vi "GetLimsTestSteps.vi"(8 "error in (no error)":errorcluster, 10 "Test-id":i32, 11 "ByteGSAPIBase in":refnum<class "ByteGSAPIBase.lvclass">) -> (0 "error out":errorcluster, 2 "Test Steps List":T1[](array[typedef]), 3 "ByteGSAPIBase out":refnum<class "ByteGSAPIBase.lvclass">)   [LabVIEW 2019, in "ByteGSWebAPI.lvlib" / "ByteGSAPIBase.lvclass"]
doc: "Get list of steps based on Test-id"
uses:
  ByteGSAPIBase.lvclass
  TypeDef/Step.ctl
  TypeDef/Asset.ctl
  ByteGSAPIBase.lvclass/ByteGSAPIBase.ctl
  <vilib>/Bytelabs/ByteREST/ByteRESTClass/ByteRESTBase/RESTBase.lvclass
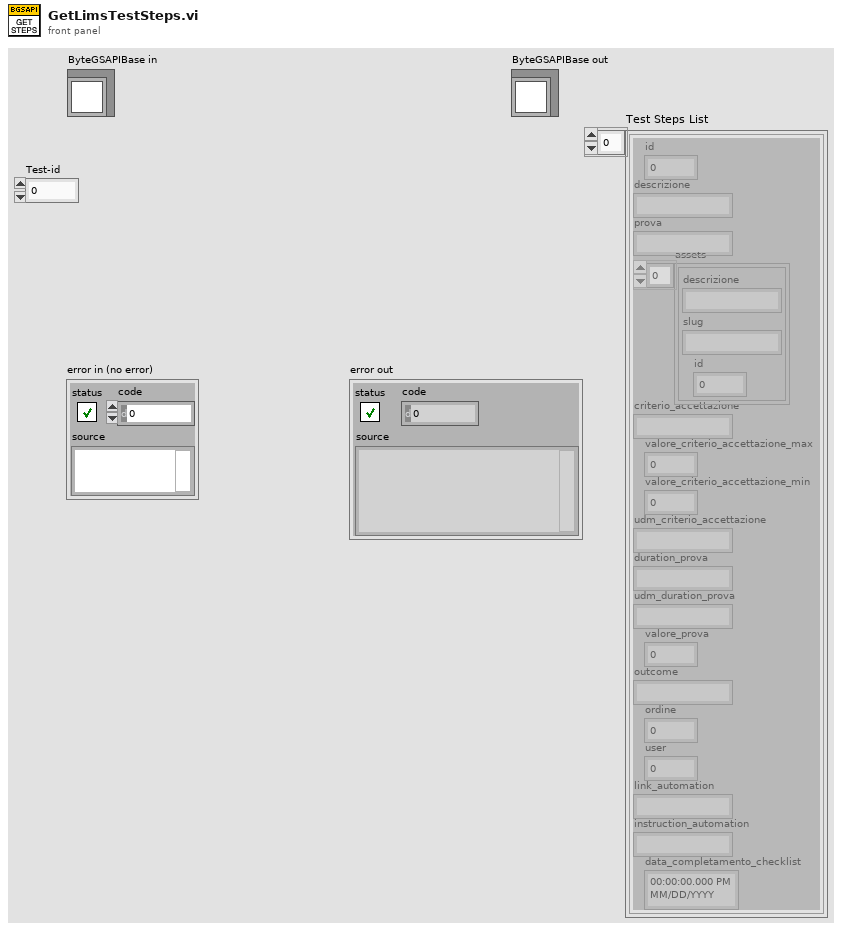
[diagram p1: front panel]
types:
  T1 = typedef "ByteGSWebAPI.lvlib/ByteGSAPIBase.lvclass/Step.ctl" = cluster{"id":i32, "descrizione":string, "prova":string, "assets":T2[], "criterio_accettazione":string, "valore_criterio_accettazione_max":dbl, "valore_criterio_accettazione_min":dbl, "udm_criterio_accettazione":string, "duration_prova":string, "udm_duration_prova":string, "valore_prova":dbl, "outcome":string, "ordine":i32, "user":i32, "link_automation":string, "instruction_automation":string, "data_completamento_checklist":timestamp}
  T2 = typedef "ByteGSWebAPI.lvlib/ByteGSAPIBase.lvclass/Asset.ctl" = cluster{"descrizione":string, "slug":string, "id":i32}
  T3 = cluster{"id":i32, "descrizione":string, "prova":string, "assets":T2[], "criterio_accettazione":string, "valore_criterio_accettazione_max":dbl, "valore_criterio_accettazione_min":dbl, "udm_criterio_accettazione":string, "duration_prova":string, "udm_duration_prova":string, "data_completamento_checklist":string, "valore_prova":dbl, "outcome":string, "ordine":i32, "user":i32, "link_automation":string, "instruction_automation":string}[]
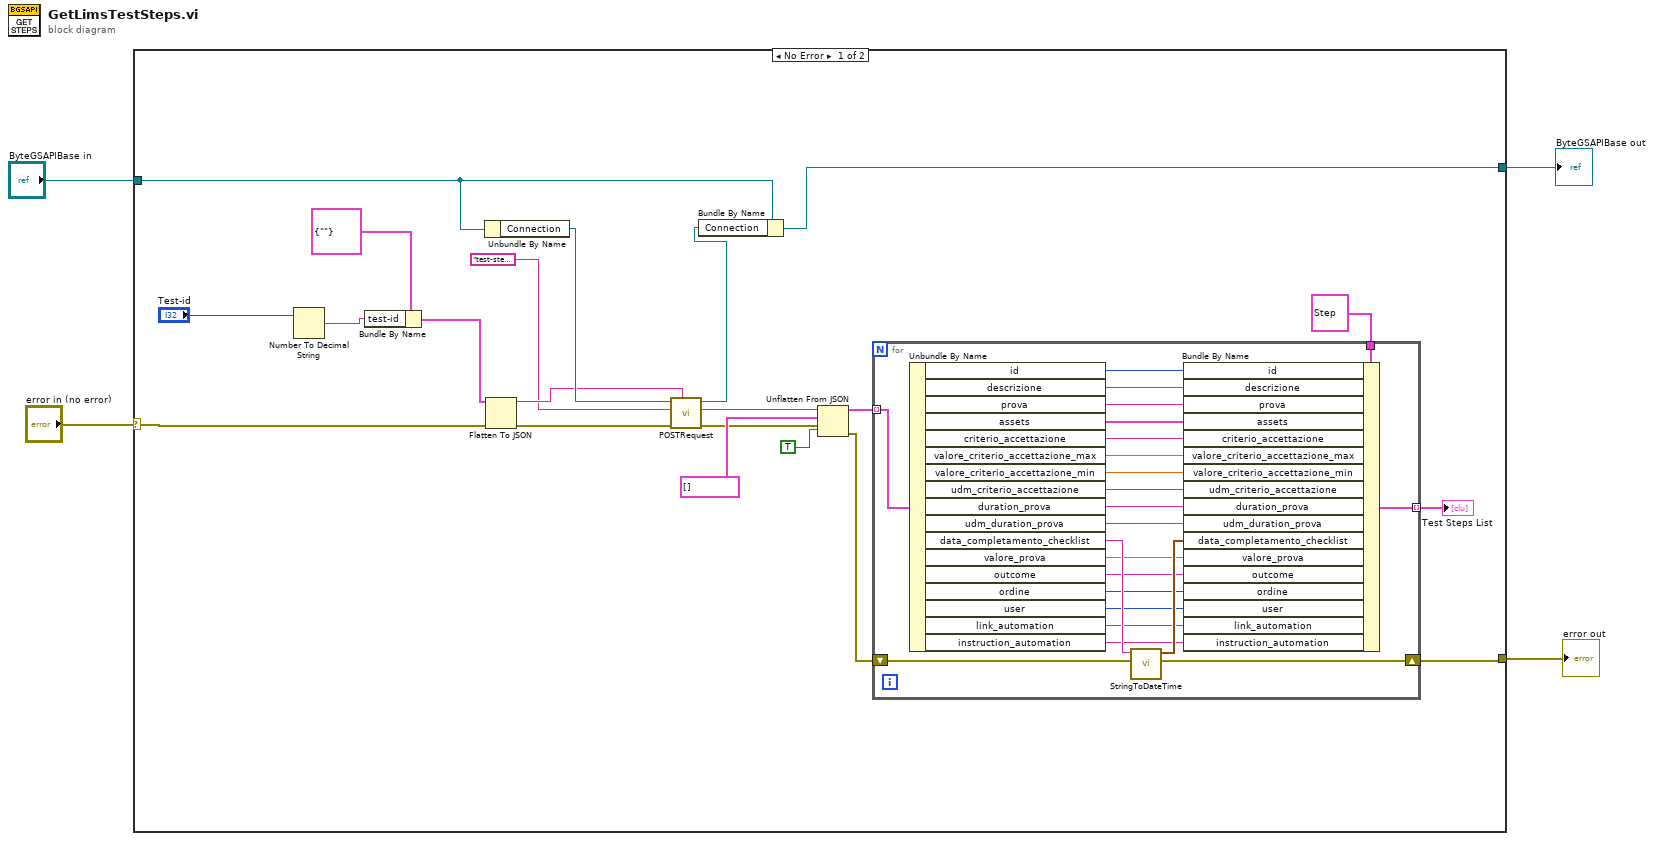
[diagram p0: block diagram]
diagram:
  n1 = case shown="No Error" "error in (no error)" {
    selector: "error in (no error)" -> [w22 w50]
    tunnel: [w7 w50] -> w3
    tunnel: [w23 w49] -> w1
    tunnel: "ByteGSAPIBase in" -> [w14 w49]
    frame No Error {
      n2 = Number To Decimal String(number="Test-id") -> (decimal integer string=w12:string)  [unwired: 1 in]
      n3 = Bundle By Name(cluster=cluster{"test-id":string} {"test-id"=""} ("Request"), "test-id"=w12) -> (w11:cluster{"test-id":string})
      n4 = Unbundle By Name(w14) -> ("Connection"=w25:refnum<class "RESTBase.lvclass">)
      n5 = Flatten To JSON(anything=w11, error in (no error)=w22) -> (JSON string=w20:string, 11:w24:errorcluster)  [unwired: 1 in]
      n6 = call-dynamic "POSTRequest.vi"("Body in"=w20, "error in (no error)"=w24, "Request"="test-step-list", "ByteRESTBase in"=w25) -> ("error out"=w18:errorcluster, "Body"=w16:string, "ByteRESTBase out"=w17:refnum<class "RESTBase.lvclass">)  [unwired: 4 in, 1 out]
      n7 = Bundle By Name(cluster=w14, "Connection"=w17) -> (w23:refnum<class "ByteGSAPIBase.lvclass">)
      n8 = Unflatten From JSON(JSON string=w16, type and defaults=T3 [], default null elements? (F)=TRUE, error in (no error)=w18) -> (value=w10:T3, error out=w8:errorcluster)  [unwired: 3 in]
      n9 = for {
        tunnel: w10 -> [w48] mode=indexing
        tunnel: T1 {"id"=0, "descrizione"="", "prova"="", "assets"=[], "criterio_accettazione"="", "valore_criterio_accettazione_max"=0.0, "valore_criterio_accettazione_min"=0.0, "udm_criterio_accettazione"="", "duration_prova"="", "udm_duration_prova"="", "valore_prova"=0.0, "outcome"="", "ordine"=0, "user"=0, "link_automation"="", "instruction_automation"="", "data_completamento_checklist"=timestamp(0 s since 1904-01-01)} -> [w47]
        shift-right: [w27] -> w7
        shift-left: w8 -> [w28]
        tunnel: [w26] -> w5 mode=indexing
        n10 = Unbundle By Name(w48) -> ("id"=w46:i32, "descrizione"=w45:string, "prova"=w44:string, "assets"=w43:T2[], "criterio_accettazione"=w42:string, "valore_criterio_accettazione_max"=w41:dbl, "valore_criterio_accettazione_min"=w40:dbl, "udm_criterio_accettazione"=w39:string, "duration_prova"=w38:string, "udm_duration_prova"=w37:string, "data_completamento_checklist"=w36:string, "valore_prova"=w34:dbl, "outcome"=w33:string, "ordine"=w32:i32, "user"=w31:i32, "link_automation"=w30:string, "instruction_automation"=w29:string)
        n11 = call "StringToDateTime.vi"("error in (no error)"=w28, "datetime string"=w36) -> ("error out"=w27:errorcluster, "timestamp"=w35:timestamp)  [unwired: 8 in]
        n12 = Bundle By Name(cluster=w47, "id"=w46, "descrizione"=w45, "prova"=w44, "assets"=w43, "criterio_accettazione"=w42, "valore_criterio_accettazione_max"=w41, "valore_criterio_accettazione_min"=w40, "udm_criterio_accettazione"=w39, "duration_prova"=w38, "udm_duration_prova"=w37, "data_completamento_checklist"=w35, "valore_prova"=w34, "outcome"=w33, "ordine"=w32, "user"=w31, "link_automation"=w30, "instruction_automation"=w29) -> (w26:T1)
      }
      "Test Steps List" <- w5
    }
    frame Error {
    }
  }
  "error out" <- w3
  "ByteGSAPIBase out" <- w1
